vi "define.vi"(8 "error in (no error)":errorcluster, 11 "TrajectoryDL110413StraightLine in":refnum<class "TrajectoryDL110420DoubleCircle.lvclass">) -> (0 "error out":errorcluster, 3 "TrajectoryDL110413StraightLine out":refnum<class "TrajectoryDL110420DoubleCircle.lvclass">)   [LabVIEW 2010, in "TrajectoryDL110420DoubleCircle.lvclass"]
doc: "modal dialog on which the user can set the trajectory parameters"
uses:
  TrajectoryDL110420DoubleCircle.lvclass
  common/xcontrols/XImage/XImage/XImage.xctl
  common/classes/ImageCollection/ImageCollection/ImageCollection.lvclass
  common/xcontrols/XImage/XImage/ROI_mode_enum.ctl
  TrajectoryDL110420DoubleCircle.lvclass/TrajectoryDL110420DoubleCircle.ctl
panel:
  in  "cancelButton":bool
  in  "okButton":bool
  in  "Tab Control":enum32{"User", "About"}(tab)
  in  "crossing parameter":dbl=5.0
  in  "number of pixels":i32
  in  "XImage":refnum<class "ImageCollection.lvclass">(xcontrol)
  # "TrajectoryDL110413StraightLine\n\nimplemented by: Dominik Langer, University of Zurich, Switzerland"
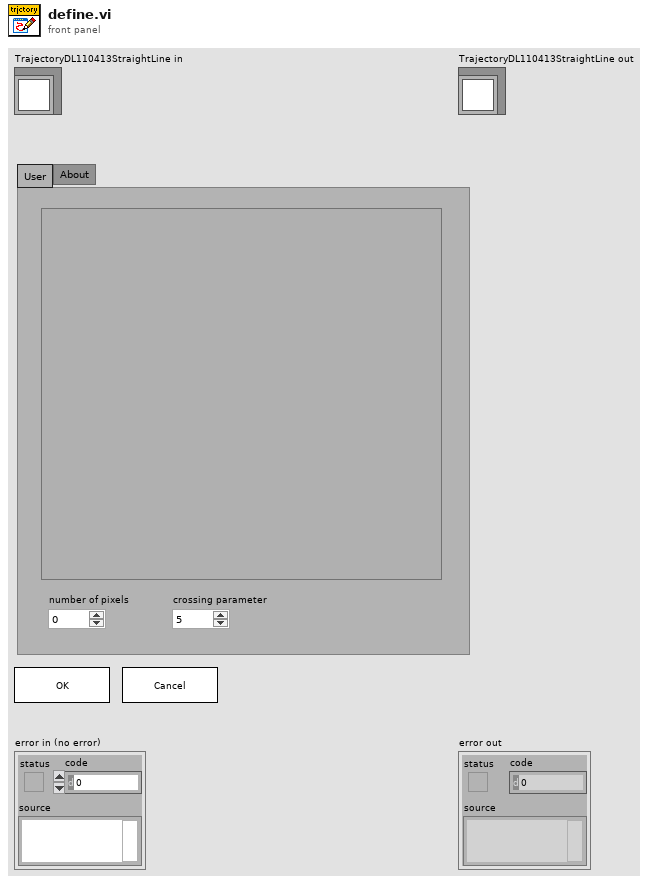
[diagram p1: front panel]
types:
  T1 = typedef "XImage.xctl/ROI_mode_enum.ctl" = enum16{"none", "IMAQROIs", "PointCollection"}
  T2 = typedef "XImage.xctl/ROImicrons_frames_cluster.ctl" = cluster{"ROI":T3[]}
  T3 = typedef "ROImicrons_cluster.ctl" = cluster{"Global Rectangle":dbl[unit][], "Contours":cluster{"Contour Type":u32, "ROI Type":u32, "Points":dbl[unit][]}[]}
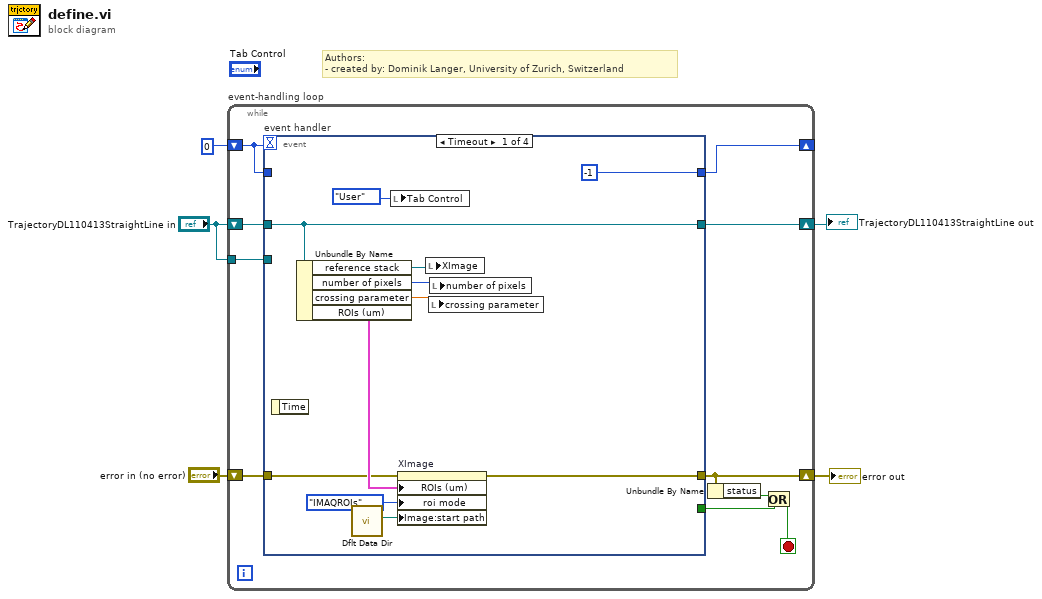
[diagram p0: block diagram]
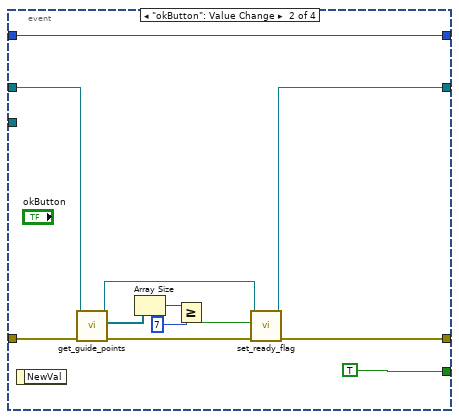
[diagram p2: hidden frame]
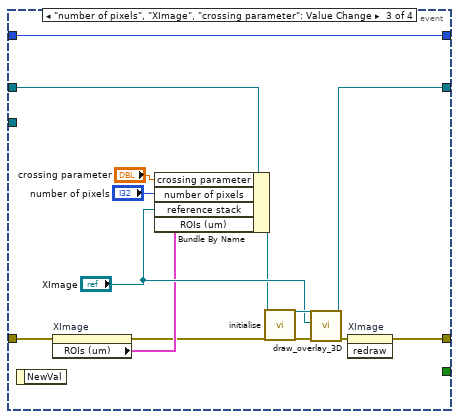
[diagram p3: hidden frame]
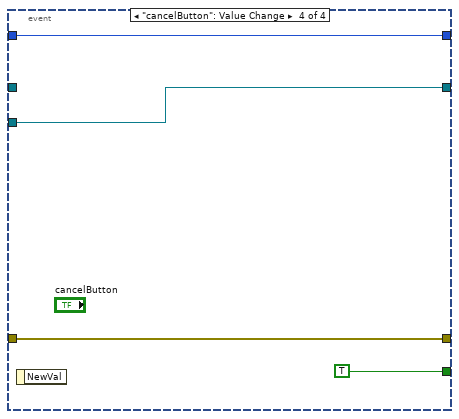
[diagram p4: hidden frame]
diagram:
  # "Authors: \n- created by: Dominik Langer, University of Zurich, Switzerland"
  n1 = while "event-handling loop" {
    shift-right: [w12] -> w4
    shift-left: "error in (no error)" -> [w15]
    shift-right: [w7] -> _
    shift-left: 0 -> [w8]
    shift-right: [w13] -> w3
    shift-left: "TrajectoryDL110413StraightLine in" -> [w14]
    tunnel: "TrajectoryDL110413StraightLine in" -> [w6]
    stop <- w9 stop-if-true
    n2 = event "event handler" shown="[0] Timeout" {
      selector: _ -> [_ _ _ _]
      dyn-events: _ -> [_ _ _ _]
      timeout: w8 -> [_ _ _ _]
      tunnel: [w20 w32 w42 w56] -> w12
      tunnel: w15 -> [w21 w31 w46 w56]
      tunnel: w14 -> [w24 w29 w50 _]
      tunnel: [w24 w34 w47 w53] -> w13
      tunnel: [_ TRUE _ TRUE] -> w10
      tunnel: [-1 w37 w52 w54] -> w7
      tunnel: w8 -> [_ w37 w52 w54]
      tunnel: w6 -> [_ _ _ w53]
      event Timeout {
        n3 = event-data() -> ()  [unwired: 1 in, 1 out]
        n4 = Unbundle By Name(w24) -> ("reference stack"=w23:refnum<class "ImageCollection.lvclass">, "number of pixels"=w19:i32, "crossing parameter"=w18:dbl, "ROIs (um)"=w22:T2)
        n5 = call <vilib>:"Dflt Data Dir.vi"() -> ("App:Default Data Directory"=w16:path)
        n6 = local write "Tab Control"(enum32{"User", "About"}."User" ("Tab Control")) -> ()
        n7 = property on="XImage" class="XImage (strict)"(error in=w21, "ROIs (um)"=w22, "roi mode"=ROI_mode_enum."IMAQROIs" ("ROI:mode"), "Image:start path"=w16) -> (error out=w20:errorcluster)  [unwired: 1 in, 1 out]
        n8 = local write "XImage"(w23) -> ()
        n9 = local write "crossing parameter"(w18) -> ()
        n10 = local write "number of pixels"(w19) -> ()
      }
      event "okButton": Value Change {
        n11 = event-data() -> ()  [unwired: 1 in, 1 out]
        n12 = call-dynamic "get_guide_points.vi"("error in (no error)"=w31, "TrajectoryDL110420DoubleCircle in"=w29) -> ("error out"=w30:errorcluster, "guide points"=w27:refnum<class "SpaceVector.lvclass">[], "TrajectoryDL110420DoubleCircle out"=w28:refnum<class "TrajectoryDL110420DoubleCircle.lvclass">)  [unwired: 7 in]
        n13 = Array Size(array=w27) -> (size(s)=w36:i32)
        n14 = Greater Or Equal?(x=w36, y=7) -> (x >= y?=w33:bool)
        n15 = call-dynamic "set_ready_flag.vi"("error in (no error)"=w30, "ready for initialisation?"=w33, "GenericTrajectory in"=w28) -> ("error out"=w32:errorcluster, "GenericTrajectory out"=w34:refnum<class "TrajectoryDL110420DoubleCircle.lvclass">)  [unwired: 7 in]
      }
      event "number of pixels", "XImage", "crossing parameter": Value Change {
        n16 = event-data() -> ()  [unwired: 1 in, 1 out]
        n17 = property on="XImage" class="XImage (strict)"(error in=w46) -> (error out=w39:errorcluster, "ROIs (um)"=w41:T2)  [unwired: 1 in, 1 out]
        n18 = Bundle By Name(cluster=w50, "crossing parameter"="crossing parameter", "number of pixels"="number of pixels", "reference stack"="XImage", "ROIs (um)"=w41) -> (w40:refnum<class "TrajectoryDL110420DoubleCircle.lvclass">)
        n19 = call-dynamic "initialise.vi"("error in (no error)"=w39, "GenericTrajectory in"=w40) -> ("error out"=w49:errorcluster, "GenericTrajectory out"=w48:refnum<class "TrajectoryDL110420DoubleCircle.lvclass">)  [unwired: 8 in]
        n20 = call-dynamic "draw_overlay_3D.vi"("error in (no error)"=w49, "ImageCollection in"="XImage", "GenericTrajectory in"=w48) -> ("error out"=w43:errorcluster, "GenericTrajectory out"=w47:refnum<class "TrajectoryDL110420DoubleCircle.lvclass">)  [unwired: 6 in, 1 out]
        n21 = invoke on="XImage" class="XImage (strict)" method="redraw"(error in=w43) -> (error out=w42:errorcluster)  [unwired: 2 in, 2 out]
      }
      event "cancelButton": Value Change {
        n22 = event-data() -> ()  [unwired: 1 in, 1 out]
      }
    }
    n23 = Unbundle By Name(w12) -> ("status"=w11:bool)
    n24 = Or(x=w11, y=w10) -> (x .or. y?=w9:bool)
  }
  "error out" <- w4
  "TrajectoryDL110413StraightLine out" <- w3
